vi "IncrementTDCVal.vi"(9 "val":i32, 10 "TDC Data":i32, 11 "Boolean":bool) -> (3 "Numeric":i32)   [LabVIEW 2014]
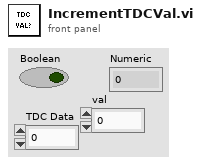
[diagram p1: front panel]
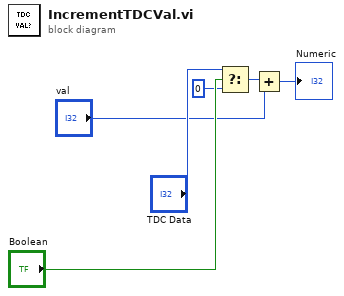
[diagram p0: block diagram]
diagram:
  n1 = Select(t="TDC Data", s="Boolean", f=0) -> (s? t:f=w4:i32)
  n2 = Add(x=w4, y="val") -> (x+y=→"Numeric":i32)
